vi "_FPGA_LasingTrigger.vi"(4 "PhaseDelay+1":u32=1, 5 "HalfPeriod+1":u32=1, 7 "ShootNum":u8=1, 8 "BypassPhaseLocking":bool, 9 "ZeroPhaseTrigger":bool, 11 "Enable_latch":bool) -> (2 "Trigger_out":bool, 3 "Lasing?":bool)   [LabVIEW 2018]
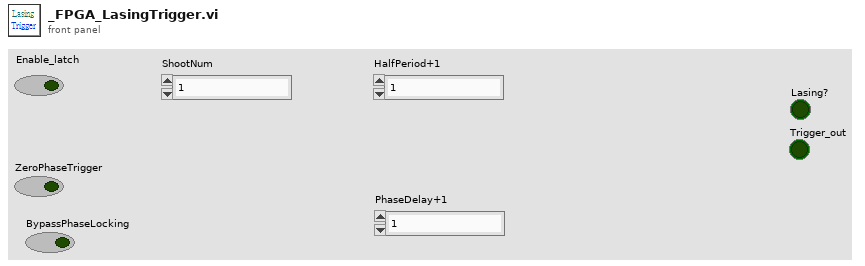
[diagram p1: front panel]
types:
  T1 = enum16{"Standby", "Load_ShootNum", "Wait_for_ZeroPhaseTrigger", "Delay", "Pulse", "Space", "ShootNum-1"}
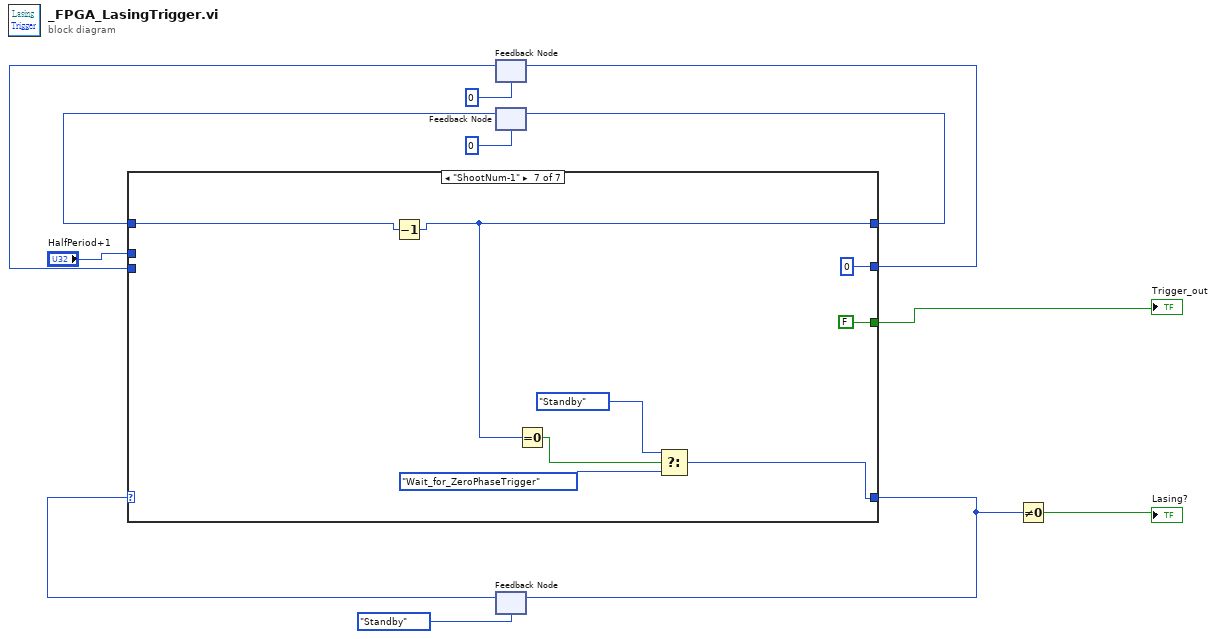
[diagram p0: block diagram]
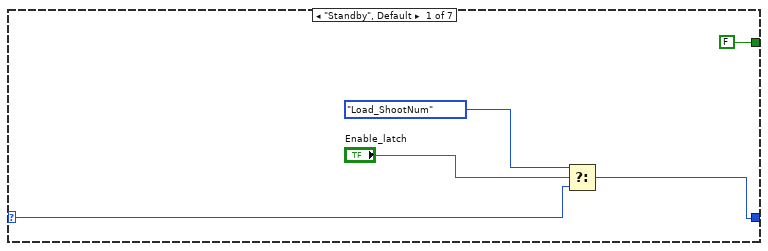
[diagram p2: hidden frame]
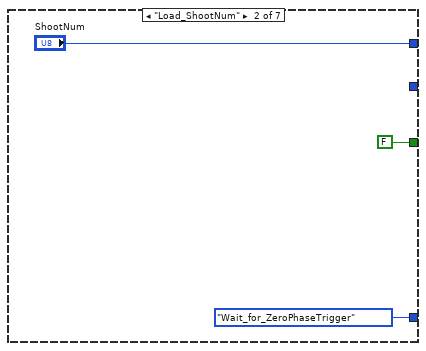
[diagram p3: hidden frame]
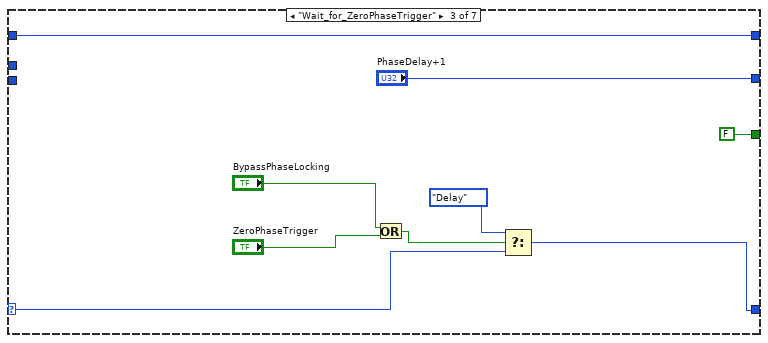
[diagram p4: hidden frame]
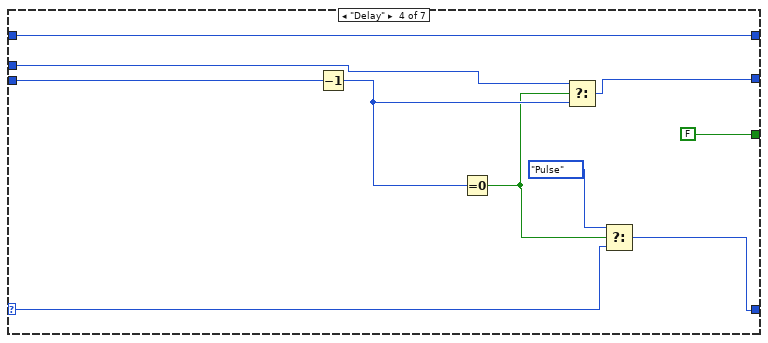
[diagram p5: hidden frame]
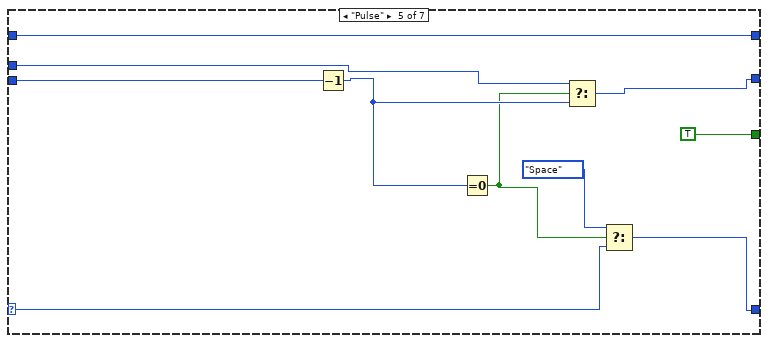
[diagram p6: hidden frame]
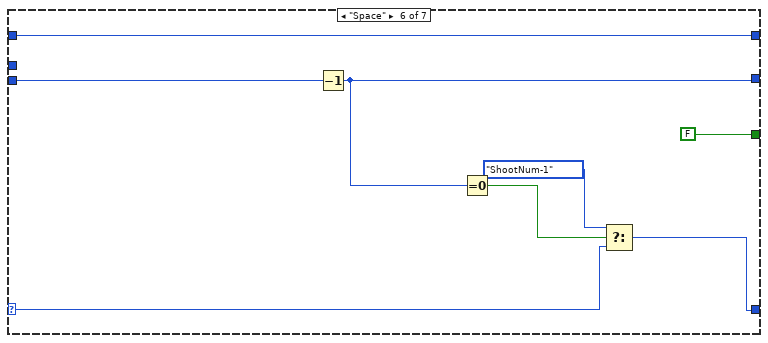
[diagram p7: hidden frame]
diagram:
  n1 = feedback #1(u32 0 ("PhaseDelay+1")) -> (w4:u32)
  n2 = feedback #2(u8 0 ("ShootNum")) -> (w10:u8)
  n3 = feedback #3(T1."Standby") -> (w12:T1)
  n4 = case shown="\"ShootNum-1\"" w12 {
    selector: w12 -> [w14 _ w25 w37 w47 w55 _]
    tunnel: [w16 T1."Wait_for_ZeroPhaseTrigger" ("f") w24 w34 w44 w52 w62] -> w7
    tunnel: [_ "ShootNum" w29 w39 w49 w57 w64] -> w11
    tunnel: w10 -> [_ _ w29 w39 w49 w57 w65]
    tunnel: [_ _ "PhaseDelay+1" w33 w43 w50 u32 0 ("Space_interval")] -> w5
    tunnel: w4 -> [_ _ _ w38 w48 w56 _]
    tunnel: [FALSE FALSE FALSE FALSE TRUE FALSE FALSE] -> w1
    tunnel: "HalfPeriod+1" -> [_ _ _ w30 w40 _ _]
    frame "Standby", Default {
      n5 = Select(t=T1."Load_ShootNum", s="Enable_latch", f=w14) -> (s? t:f=w16:T1)
    }
    frame "Load_ShootNum" {
    }
    frame "Wait_for_ZeroPhaseTrigger" {
      n6 = Or(x="BypassPhaseLocking", y="ZeroPhaseTrigger") -> (x .or. y?=w27:bool)
      n7 = Select(t=T1."Delay", s=w27, f=w25) -> (s? t:f=w24:T1)
    }
    frame "Delay" {
      n8 = Decrement(x=w38) -> (x-1=w32:u32)
      n9 = Equal To 0?(x=w32) -> (x = 0?=w31:bool)
      n10 = Select(t=w30, s=w31, f=w32) -> (s? t:f=w33:u32)
      n11 = Select(t=T1."Pulse", s=w31, f=w37) -> (s? t:f=w34:T1)
    }
    frame "Pulse" {
      n12 = Decrement(x=w48) -> (x-1=w42:u32)
      n13 = Equal To 0?(x=w42) -> (x = 0?=w41:bool)
      n14 = Select(t=w40, s=w41, f=w42) -> (s? t:f=w43:u32)
      n15 = Select(t=T1."Space", s=w41, f=w47) -> (s? t:f=w44:T1)
    }
    frame "Space" {
      n16 = Decrement(x=w56) -> (x-1=w50:u32)
      n17 = Equal To 0?(x=w50) -> (x = 0?=w51:bool)
      n18 = Select(t=T1."ShootNum-1", s=w51, f=w55) -> (s? t:f=w52:T1)
    }
    frame "ShootNum-1" {
      n19 = Decrement(x=w65) -> (x-1=w64:u8)
      n20 = Equal To 0?(x=w64) -> (x = 0?=w63:bool)
      n21 = Select(t=T1."Standby", s=w63, f=T1."Wait_for_ZeroPhaseTrigger") -> (s? t:f=w62:T1)
    }
  }
  "Trigger_out" <- w1
  n22 = feedback-in #1(w5) -> ()
  n23 = feedback-in #2(w11) -> ()
  n24 = feedback-in #3(w7) -> ()
  n25 = Not Equal To 0?(x=w7) -> (x != 0?=→"Lasing?":bool)
